vi "Delete TDMS channel.vi"(8 "Error In":errorcluster, 9 "Channel":string, 10 "Group":string="Untitled", 11 "Source Path":path) -> (0 "Error Out":errorcluster, 3 "Source Path out":path)   [LabVIEW 2015]
uses:
  <vilib>/Platform/storage/utility/usiTDMTDMS.ctl
  <vilib>/Platform/storage/lvStorage.llb/_openFunction.ctl
  <vilib>/Platform/storage/lvStorage.llb/_openStorageWithRootAutoDetect.vi
  <vilib>/Platform/storage/lvStorage.llb/xStorage/xStorageSupp/ErrorOut.vi
  <vilib>/Platform/storage/Storage.llb/__loadPropString.vi
  <vilib>/Platform/storage/Storage.llb/__loadPropTime.vi
  <vilib>/Platform/storage/Storage.llb/__loadPropRefList.vi
  <vilib>/Platform/storage/lvStorage.llb/_loadDDT.vi
  <vilib>/Platform/storage/lvStorage.llb/Delete Channel.vi
  <vilib>/Platform/storage/Storage.llb/Get Object Info.vi
  <vilib>/Platform/storage/Storage.llb/__closeStorageFromObject.vi
  <vilib>/Platform/storage/lvStorage.llb/xStorage/Open Data Storage/Open Data Storage.xnode
  <vilib>/Platform/storage/lvStorage.llb/xStorage/Get Properties/Get Properties.xnode
  <vilib>/Platform/storage/lvStorage.llb/xStorage/Close Data Storage/Close Data Storage.xnode
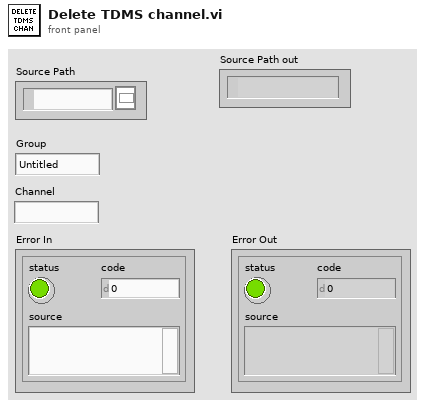
[diagram p1: front panel]
types:
  T1 = typedef "usiTDMTDMS.ctl" = enum16{"TDM", "TDMS"}
  T2 = typedef "_openFunction.ctl" = enum16{"open", "open or create", "create or replace", "create", "open (read only)"}
  T3 = enum16{"UPDATE", "READ", "QUERY", "CREATE CHILD", "CREATE", "CONNECT", "DISCONNECT"}
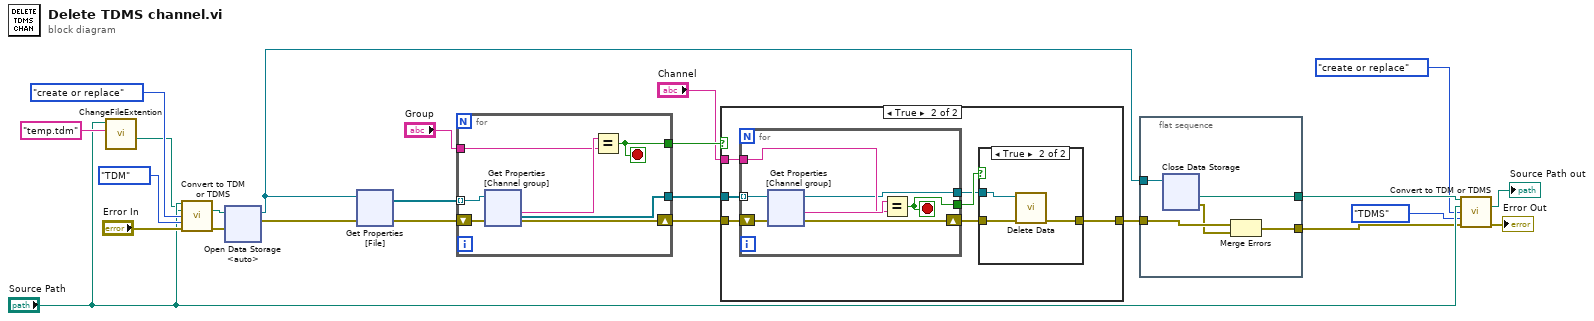
[diagram p0: block diagram]
diagram:
  n1 = call "ChangeFileExtention.vi"("New Extention"="temp.tdm", "Path"="Source Path") -> ("Path with new extension"=w2:path)  [unwired: 5 in, 4 out]
  n2 = call <vilib>:"Convert to TDM or TDMS.vi"("source file path"="Source Path", "target file path"=w2, "target file operation (3:create)"=_openFunction."create or replace", "target file format (TDMS)"=usiTDMTDMS."TDM", "error in (no error)"="Error In") -> ("target file path out"=w20:path, "error out"=w19:errorcluster)  [unwired: 7 in, 2 out]
  n3 = xnode "Open Data Storage\n<auto>"("file path"=w20, "error in (no error)"=w19) -> ("storage refnum (file)"=w10:refnum<k20>, "error out"=w13:errorcluster)  [unwired: 3 in, 1 out]
  n4 = xnode "Get Properties\n[File]"("storage refnum (file)"=w10, "error in"=w13) -> ("error out"=w12:errorcluster, "storage refnums (channel group)"=w18:refnum<k20>[])  [unwired: 6 out]
  n5 = for {
    tunnel: w18 -> [w31] mode=indexing
    tunnel: "Group" -> [w29]
    tunnel: [w28] -> w16
    tunnel: [w27] -> w15
    shift-right: [w25] -> w11
    shift-left: w12 -> [w26]
    stop <- w28 stop-if-true
    n6 = xnode "Get Properties\n[Channel group]"("storage refnum (channel group)"=w31, "error in"=w26) -> ("error out"=w25:errorcluster, "Name"=w30:string, "storage refnums (channel)"=w27:refnum<k20>[])  [unwired: 2 out]
    n7 = Equal?(x=w30, y=w29) -> (x = y?=w28:bool)
  }
  n8 = case shown="True" w16 {
    tunnel: w15 -> [_ w55]
    tunnel: "Channel" -> [_ w54]
    tunnel: w11 -> [w48 w51]
    tunnel: [w48 w49] -> w9
    frame False {
    }
    frame True {
      n9 = for {
        tunnel: w55 -> [w66] mode=indexing
        tunnel: w54 -> [w64]
        tunnel: [w63] -> w53
        tunnel: [w62] -> w52
        shift-right: [w60] -> w50
        shift-left: w51 -> [w61]
        stop <- w63 stop-if-true
        n10 = xnode "Get Properties\n[Channel group]"("storage refnum (channel)"=w66, "error in"=w61) -> ("storage refnum (channel) out"=w62:refnum<k20>, "error out"=w60:errorcluster, "Name"=w65:string)  [unwired: 2 in, 2 out]
        n11 = Equal?(x=w65, y=w64) -> (x = y?=w63:bool)
      }
      n12 = case shown="True" w53 {
        tunnel: w52 -> [_ w59]
        tunnel: w50 -> [w56 w58]
        tunnel: [w56 w57] -> w49
        frame False {
        }
        frame True {
          n13 = call-poly <vilib>:"Delete Data.vi"("error in (no error)"=w58, "storage refnum (channel)"=w59) -> ("error out"=w57:errorcluster)  [unwired: 5 in]
        }
      }
    }
  }
  n14 = flat-sequence {
    tunnel: w10 -> [w88]
    tunnel: w9 -> [w87]
    tunnel: [w85] -> w8
    tunnel: [w84] -> w5
    frame #0 {
      n15 = xnode "Close Data Storage"("storage refnum (file)"=w88) -> ("file path"=w85:path, "error out"=w86:errorcluster)  [unwired: 1 in]
      n16 = Merge Errors(w87, w86) -> (w84:errorcluster)
    }
  }
  n17 = call <vilib>:"Convert to TDM or TDMS.vi"("source file path"=w8, "target file path"="Source Path", "target file operation (3:create)"=_openFunction."create or replace", "target file format (TDMS)"=usiTDMTDMS."TDMS", "error in (no error)"=w5) -> ("target file path out"=→"Source Path out":path, "error out"=→"Error Out":errorcluster)  [unwired: 7 in, 2 out]
